vi "randomNumberTimer.vi"() -> ()   [LabVIEW 2023]
uses:
  <vilib>/numeric/Random Number (Range) DBL.vi
panel:
  out "time spent":u32
  out "Iterations":i32
  out "Random number":dbl
  out "x = y?":bool
  in  "Target Number (0-100)":dbl
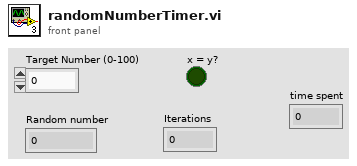
[diagram p1: front panel]
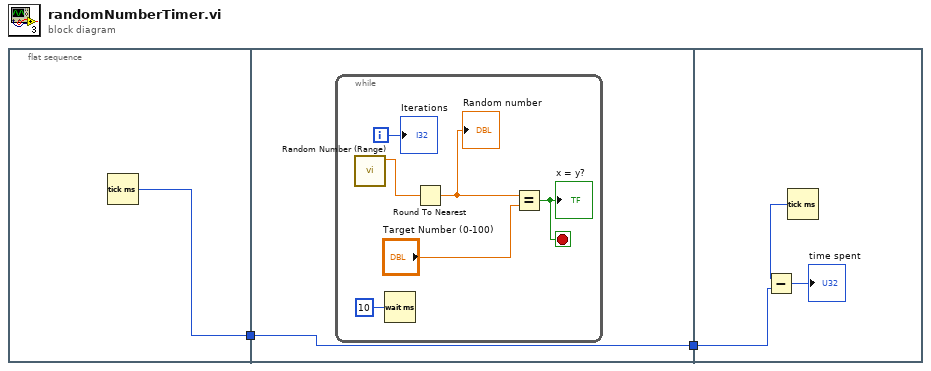
[diagram p0: block diagram]
diagram:
  n1 = flat-sequence {
    tunnel: [w3] -> w1
    tunnel: [w4] -> w2
    tunnel: w1 -> [w4]
    tunnel: w2 -> [w13]
    frame #0 {
      n2 = Tick Count (ms)() -> (millisecond timer value=w3:u32)
    }
    frame #1 {
      n3 = while {
        i -> [w6]
        stop <- w7 stop-if-true
        n4 = call-poly <vilib>:"Random Number (Range).vi"() -> ("number"=w10:dbl)  [unwired: 11 in]
        n5 = Wait (ms)(milliseconds to wait=u32 10) -> ()  [unwired: 1 out]
        n6 = Round To Nearest(number=w10) -> (nearest integer value=w8:dbl)
        "Random number" <- w8
        n7 = Equal?(x=w8, y="Target Number (0-100)") -> (x = y?=w7:bool)
        "x = y?" <- w7
        "Iterations" <- w6
      }
    }
    frame #2 {
      n8 = Tick Count (ms)() -> (millisecond timer value=w12:u32)
      n9 = Subtract(x=w12, y=w13) -> (x-y=→"time spent":u32)
    }
  }
